vi "DetermineDecimation.vi"(8 "error in (no error)":errorcluster, 10 "input buffer size":i32, 11 "display width":i32) -> (0 "error out":errorcluster, 1 "no decimation?":bool, 2 "output buffer size":i32, 3 "decimation\nfactor":i32)   [LabVIEW 2015]
doc: "This VI calculates the decimation factor and display buffer size for a max/min decimation using the <B>sfpCore Specified Max Min Decimate Ixx 1D Array</B> VIs."
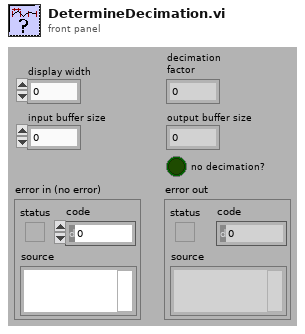
[diagram p1: front panel]
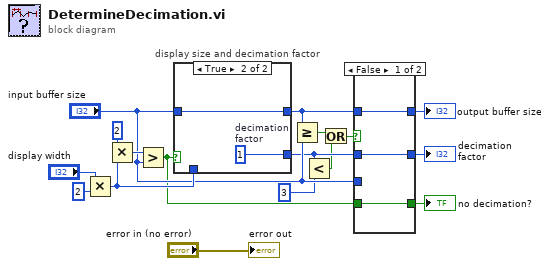
[diagram p0: block diagram]
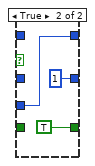
[diagram p2: hidden frame]
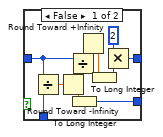
[diagram p3: hidden frame]
diagram:
  n1 = Multiply(x="display width", y=2) -> (x*y=w17:i32)
  n2 = Multiply(x=2, y=w17) -> (x*y=w16:i32)
  n3 = Greater?(x=w16, y="input buffer size") -> (0:w1:bool)
  n4 = case "display size and decimation factor" shown="True" w1 {
    tunnel: "input buffer size" -> [w18 w29]
    tunnel: w17 -> [w27 _]
    tunnel: [w20 w29] -> w10
    tunnel: [w25 w28] -> w6
    frame False {
      n5 = Divide(x=w18, y=w27) -> (x/y=w26:dbl)
      n6 = Round Toward -Infinity(1:w26) -> (0:w24:dbl)
      n7 = Divide(x=w18, y=w24) -> (x/y=w23:dbl)
      n8 = To Long Integer(number=w24) -> (32bit integer=w25:i32)
      n9 = Round Toward +Infinity(x=w23) -> (ceil(x): smallest int >= x=w22:dbl)
      n10 = To Long Integer(number=w22) -> (32bit integer=w21:i32)
      n11 = Multiply(x=2, y=w21) -> (x*y=w20:i32)
    }
    frame True {
      w28 = 1  # decimation factor
    }
  }
  n12 = Greater Or Equal?(x=w10, y="input buffer size") -> (x >= y?=w3:bool)
  n13 = Less?(x=w6, y=3) -> (x < y?=w2:bool)
  n14 = Or(x=w3, y=w2) -> (x .or. y?=w4:bool)
  n15 = case shown="False" w4 {
    tunnel: "input buffer size" -> [_ w33]
    tunnel: w10 -> [w32 _]
    tunnel: [w32 w33] -> w9
    tunnel: w6 -> [w31 _]
    tunnel: [w31 1 ("decimation\nfactor")] -> w8
    tunnel: w1 -> [w30 _]
    tunnel: [w30 TRUE] -> w7
    frame False {
    }
    frame True {
    }
  }
  "decimation\nfactor" <- w8
  "output buffer size" <- w9
  "no decimation?" <- w7
  "error out" <- "error in (no error)"
